vi "display language.vi"(6 "Language":T1, 8 "error in":errorcluster, 10 "Language data":T2=[{"Label.Text"="Quit", "Control Type"=0, "Numeric"=0.0, "Array"=[], "status"=FALSE, "Str Array"=[], "String"="", "unit"=""}, {"Label.Text"="Tab Control", "Control Type"=0, "Numeric"=0.0, "Array"=[], "status"=FALSE, "Str Array"=[], "String"="", "unit"=""}, {"Label.Text"="Help Button", "Control Type"=0, "Numeric"=0.0, "Array"=[], "status"=FALSE, "Str Array"=[], "String"="", "unit"=""}, {"Label.Text"="Logon", "Control Type"=0, "Numeric"=0.0, "Array"=[], "status"=FALSE, "Str Array"=[], "String"="", "unit"=""}, {"Label.Text"="Project List", "Control Type"=0, "Numeric"=0.0, "Array"=[], "status"=FALSE, "Str Array"=[], "String"="", "unit"=""}, {"Label.Text"="Project commands", "Control Type"=0, "Numeric"=0.0, "Array"=[], "status"=FALSE, "Str Array"=[], "String"="", "unit"=""}, {"Label.Text"="Log off", "Control Type"=0, "Numeric"=0.0, "Array"=[], "status"=FALSE, "Str Array"=[], "String"="", "unit"=""}, {"Label.Text"="Design Plant", "Control Type"=0, "Numeric"=0.0, "Array"=[], "status"=FALSE, "Str Array"=[], "String"="", "unit"=""}, {"Label.Text"="Project Info label", "Control Type"=0, "Numeric"=0.0, "Array"=[], "status"=FALSE, "Str Array"=[], "String"="", "unit"=""}, {"Label.Text"="Design Inputs Label", "Control Type"=0, "Numeric"=0.0, "Array"=[], "status"=FALSE, "Str Array"=[], "String"="", "unit"=""}, {"Label.Text"="MSG Design sent precity", "Control Type"=0, "Numeric"=0.0, "Array"=[], "status"=FALSE, "Str Array"=[], "String"="", "unit"=""}, {"Label.Text"="MSG Design sent postcity", "Control Type"=0, "Numeric"=0.0, "Array"=[], "status"=FALSE, "Str Array"=[], "String"="", "unit"=""}, {"Label.Text"="MSG Server unavailable", "Control Type"=0, "Numeric"=0.0, "Array"=[], "status"=FALSE, "Str Array"=[], "String"="", "unit"=""}, {"Label.Text"="Quit now", "Control Type"=0, "Numeric"=0.0, "Array"=[], "status"=FALSE, "Str Array"=[], "String"="", "unit"=""}, {"Label.Text"="Project Info", "Control Type"=0, "Numeric"=0.0, "Array"=[], "status"=FALSE, "Str Array"=[], "String"="", "unit"=""}, {"Label.Text"="Project Name", "Control Type"=0, "Numeric"=0.0, "Array"=[], "status"=FALSE, "Str Array"=[], "String"="", "unit"=""}, {"Label.Text"="City", "Control Type"=0, "Numeric"=0.0, "Array"=[], "status"=FALSE, "Str Array"=[], "String"="", "unit"=""}, {"Label.Text"="State", "Control Type"=0, "Numeric"=0.0, "Array"=[], "status"=FALSE, "Str Array"=[], "String"="", "unit"=""}, {"Label.Text"="Country", "Control Type"=0, "Numeric"=0.0, "Array"=[], "status"=FALSE, "Str Array"=[], "String"="", "unit"=""}, {"Label.Text"="Notes", "Control Type"=0, "Numeric"=0.0, "Array"=[], "status"=FALSE, "Str Array"=[], "String"="", "unit"=""}, {"Label.Text"="User Information", "Control Type"=0, "Numeric"=0.0, "Array"=[], "status"=FALSE, "Str Array"=[], "String"="", "unit"=""}, {"Label.Text"="First Name", "Control Type"=0, "Numeric"=0.0, "Array"=[], "status"=FALSE, "Str Array"=[], "String"="", "unit"=""}, {"Label.Text"="Last Name", "Control Type"=0, "Numeric"=0.0, "Array"=[], "status"=FALSE, "Str Array"=[], "String"="", "unit"=""}, {"Label.Text"="Email Address", "Control Type"=0, "Numeric"=0.0, "Array"=[], "status"=FALSE, "Str Array"=[], "String"="", "unit"=""}, {"Label.Text"="Organization", "Control Type"=0, "Numeric"=0.0, "Array"=[], "status"=FALSE, "Str Array"=[], "String"="", "unit"=""}, {"Label.Text"="Language", "Control Type"=0, "Numeric"=0.0, "Array"=[], "status"=FALSE, "Str Array"=[], "String"="", "unit"=""}, {"Label.Text"="AutoCAD File Type", "Control Type"=0, "Numeric"=0.0, "Array"=[], "status"=FALSE, "Str Array"=[], "String"="", "unit"=""}, {"Label.Text"="Project date", "Control Type"=0, "Numeric"=0.0, "Array"=[], "status"=FALSE, "Str Array"=[], "String"="", "unit"=""}, {"Label.Text"="Design Inputs", "Control Type"=0, "Numeric"=0.0, "Array"=[], "status"=FALSE, "Str Array"=[], "String"="", "unit"=""}, {"Label.Text"="Q.Plant", "Control Type"=0, "Numeric"=0.0, "Array"=[], "status"=FALSE, "Str Array"=[], "String"="", "unit"=""}, {"Label.Text"="C.CoagDoseMax", "Control Type"=0, "Numeric"=0.0, "Array"=[], "status"=FALSE, "Str Array"=[], "String"="", "unit"=""}, {"Label.Text"="C.CoagStock", "Control Type"=0, "Numeric"=0.0, "Array"=[], "status"=FALSE, "Str Array"=[], "String"="", "unit"=""}, {"Label.Text"="Ti.CoagStock", "Control Type"=0, "Numeric"=0.0, "Array"=[], "status"=FALSE, "Str Array"=[], "String"="", "unit"=""}, {"Label.Text"="EN.DrillSeries", "Control Type"=0, "Numeric"=0.0, "Array"=[], "status"=FALSE, "Str Array"=[], "String"="", "unit"=""}, {"Label.Text"="EN.TubeSeries", "Control Type"=0, "Numeric"=0.0, "Array"=[], "status"=FALSE, "Str Array"=[], "String"="", "unit"=""}, {"Label.Text"="EN.PipeSeries", "Control Type"=0, "Numeric"=0.0, "Array"=[], "status"=FALSE, "Str Array"=[], "String"="", "unit"=""}, {"Label.Text"="N.SedTanks", "Control Type"=0, "Numeric"=0.0, "Array"=[], "status"=FALSE, "Str Array"=[], "String"="", "unit"=""}, {"Label.Text"="N.SedBaysEst", "Control Type"=0, "Numeric"=0.0, "Array"=[], "status"=FALSE, "Str Array"=[], "String"="", "unit"=""}, {"Label.Text"="W.SedPlate", "Control Type"=0, "Numeric"=0.0, "Array"=[], "status"=FALSE, "Str Array"=[], "String"="", "unit"=""}, {"Label.Text"="L.SedPlateSheet", "Control Type"=0, "Numeric"=0.0, "Array"=[], "status"=FALSE, "Str Array"=[], "String"="", "unit"=""}, {"Label.Text"="T.SedPlate", "Control Type"=0, "Numeric"=0.0, "Array"=[], "status"=FALSE, "Str Array"=[], "String"="", "unit"=""}, {"Label.Text"="T.PlantWall", "Control Type"=0, "Numeric"=0.0, "Array"=[], "status"=FALSE, "Str Array"=[], "String"="", "unit"=""}, {"Label.Text"="H.FlocOption", "Control Type"=0, "Numeric"=0.0, "Array"=[], "status"=FALSE, "Str Array"=[], "String"="", "unit"=""}, {"Label.Text"="T.FlocBaffleRigidH", "Control Type"=0, "Numeric"=0.0, "Array"=[], "status"=FALSE, "Str Array"=[], "String"="", "unit"=""}, {"Label.Text"="T.ConcreteMin", "Control Type"=0, "Numeric"=0.0, "Array"=[], "status"=FALSE, "Str Array"=[], "String"="", "unit"=""}, {"Label.Text"="T.SedWeir", "Control Type"=0, "Numeric"=0.0, "Array"=[], "status"=FALSE, "Str Array"=[], "String"="", "unit"=""}, {"Label.Text"="T.FlocBaffleRigidV", "Control Type"=0, "Numeric"=0.0, "Array"=[], "status"=FALSE, "Str Array"=[], "String"="", "unit"=""}, {"Label.Text"="error out", "Control Type"=0, "Numeric"=0.0, "Array"=[], "status"=FALSE, "Str Array"=[], "String"="", "unit"=""}, {"Label.Text"="status", "Control Type"=0, "Numeric"=0.0, "Array"=[], "status"=FALSE, "Str Array"=[], "String"="", "unit"=""}, {"Label.Text"="code", "Control Type"=0, "Numeric"=0.0, "Array"=[], "status"=FALSE, "Str Array"=[], "String"="", "unit"=""}, {"Label.Text"="source", "Control Type"=0, "Numeric"=0.0, "Array"=[], "status"=FALSE, "Str Array"=[], "String"="", "unit"=""}, {"Label.Text"="File List", "Control Type"=0, "Numeric"=0.0, "Array"=[], "status"=FALSE, "Str Array"=[], "String"="", "unit"=""}, {"Label.Text"="Translate", "Control Type"=0, "Numeric"=0.0, "Array"=[], "status"=FALSE, "Str Array"=[], "String"="", "unit"=""}, {"Label.Text"="CheckOut ADT", "Control Type"=0, "Numeric"=0.0, "Array"=[], "status"=FALSE, "Str Array"=[], "String"="", "unit"=""}, {"Label.Text"="ADT version", "Control Type"=0, "Numeric"=0.0, "Array"=[], "status"=FALSE, "Str Array"=[], "String"="", "unit"=""}, {"Label.Text"="Choose Server", "Control Type"=0, "Numeric"=0.0, "Array"=[], "status"=FALSE, "Str Array"=[], "String"="", "unit"=""}, {"Label.Text"="design server", "Control Type"=0, "Numeric"=0.0, "Array"=[], "status"=FALSE, "Str Array"=[], "String"="", "unit"=""}, {"Label.Text"="Restart ADT", "Control Type"=0, "Numeric"=0.0, "Array"=[], "status"=FALSE, "Str Array"=[], "String"="", "unit"=""}, {"Label.Text"="Create New Project", "Control Type"=0, "Numeric"=0.0, "Array"=[], "status"=FALSE, "Str Array"=[], "String"="", "unit"=""}, {"Label.Text"="Edit Project", "Control Type"=0, "Numeric"=0.0, "Array"=[], "status"=FALSE, "Str Array"=[], "String"="", "unit"=""}, {"Label.Text"="Delete Project", "Control Type"=0, "Numeric"=0.0, "Array"=[], "status"=FALSE, "Str Array"=[], "String"="", "unit"=""}, {"Label.Text"="Valid User Options", "Control Type"=0, "Numeric"=0.0, "Array"=[], "status"=FALSE, "Str Array"=[], "String"="", "unit"=""}, {"Label.Text"="Okay Button", "Control Type"=0, "Numeric"=0.0, "Array"=[], "status"=FALSE, "Str Array"=[], "String"="", "unit"=""}, {"Label.Text"="logon status", "Control Type"=0, "Numeric"=0.0, "Array"=[], "status"=FALSE, "Str Array"=[], "String"="", "unit"=""}, {"Label.Text"="valid user", "Control Type"=0, "Numeric"=0.0, "Array"=[], "status"=FALSE, "Str Array"=[], "String"="", "unit"=""}, {"Label.Text"="User Information out", "Control Type"=0, "Numeric"=0.0, "Array"=[], "status"=FALSE, "Str Array"=[], "String"="", "unit"=""}, {"Label.Text"="Cancel Button", "Control Type"=0, "Numeric"=0.0, "Array"=[], "status"=FALSE, "Str Array"=[], "String"="", "unit"=""}, {"Label.Text"="User Index out", "Control Type"=0, "Numeric"=0.0, "Array"=[], "status"=FALSE, "Str Array"=[], "String"="", "unit"=""}, {"Label.Text"="User Index in", "Control Type"=0, "Numeric"=0.0, "Array"=[], "status"=FALSE, "Str Array"=[], "String"="", "unit"=""}, {"Label.Text"="New Account", "Control Type"=0, "Numeric"=0.0, "Array"=[], "status"=FALSE, "Str Array"=[], "String"="", "unit"=""}, {"Label.Text"="Update User Info", "Control Type"=0, "Numeric"=0.0, "Array"=[], "status"=FALSE, "Str Array"=[], "String"="", "unit"=""}, {"Label.Text"="Language Data", "Control Type"=0, "Numeric"=0.0, "Array"=[], "status"=FALSE, "Str Array"=[], "String"="", "unit"=""}, {"Label.Text"="OK Button", "Control Type"=0, "Numeric"=0.0, "Array"=[], "status"=FALSE, "Str Array"=[], "String"="", "unit"=""}, {"Label.Text"="Language Data out", "Control Type"=0, "Numeric"=0.0, "Array"=[], "status"=FALSE, "Str Array"=[], "String"="", "unit"=""}, {"Label.Text"="updated", "Control Type"=0, "Numeric"=0.0, "Array"=[], "status"=FALSE, "Str Array"=[], "String"="", "unit"=""}, {"Label.Text"="Table Control", "Control Type"=0, "Numeric"=0.0, "Array"=[], "status"=FALSE, "Str Array"=[], "String"="", "unit"=""}, {"Label.Text"="Load from VNG", "Control Type"=0, "Numeric"=0.0, "Array"=[], "status"=FALSE, "Str Array"=[], "String"="", "unit"=""}, {"Label.Text"="Design Inputs out", "Control Type"=0, "Numeric"=0.0, "Array"=[], "status"=FALSE, "Str Array"=[], "String"="", "unit"=""}, {"Label.Text"="Project Info out", "Control Type"=0, "Numeric"=0.0, "Array"=[], "status"=FALSE, "Str Array"=[], "String"="", "unit"=""}, {"Label.Text"="canceled", "Control Type"=0, "Numeric"=0.0, "Array"=[], "status"=FALSE, "Str Array"=[], "String"="", "unit"=""}, {"Label.Text"="Reset to Default", "Control Type"=0, "Numeric"=0.0, "Array"=[], "status"=FALSE, "Str Array"=[], "String"="", "unit"=""}, {"Label.Text"="Basic Inputs", "Control Type"=0, "Numeric"=0.0, "Array"=[], "status"=FALSE, "Str Array"=[], "String"="", "unit"=""}, {"Label.Text"="Floc tank depth controls", "Control Type"=0, "Numeric"=0.0, "Array"=[], "status"=FALSE, "Str Array"=[], "String"="", "unit"=""}, {"Label.Text"="HW.FlocEnd", "Control Type"=0, "Numeric"=0.0, "Array"=[], "status"=FALSE, "Str Array"=[], "String"="", "unit"=""}, {"Label.Text"="HW.FlocEndDepth", "Control Type"=0, "Numeric"=0.0, "Array"=[], "status"=FALSE, "Str Array"=[], "String"="", "unit"=""}, {"Label.Text"="Language data", "Control Type"=0, "Numeric"=0.0, "Array"=[], "status"=FALSE, "Str Array"=[], "String"="", "unit"=""}, {"Label.Text"="error in", "Control Type"=0, "Numeric"=0.0, "Array"=[], "status"=FALSE, "Str Array"=[], "String"="", "unit"=""}, {"Label.Text"="VI controls", "Control Type"=0, "Numeric"=0.0, "Array"=[], "status"=FALSE, "Str Array"=[], "String"="", "unit"=""}, {"Label.Text"="Progress bar", "Control Type"=0, "Numeric"=0.0, "Array"=[], "status"=FALSE, "Str Array"=[], "String"="", "unit"=""}], 11 "VI controls":refnum<vi>[](array[refnum])) -> (0 "error out":errorcluster)   [LabVIEW 2015, in "AguaClara Library.lvlib"]
uses:
  AguaClara Library.lvlib
  Language.ctl
  Variable cluster.ctl
panel:
  out "Control labels":string[](array[string])
  out "Progress bar":dbl(slide) caption="Traduciendo" max=314.0 scale=0.0..1.0
  in  "Cancel Button":bool caption="Cancelar"
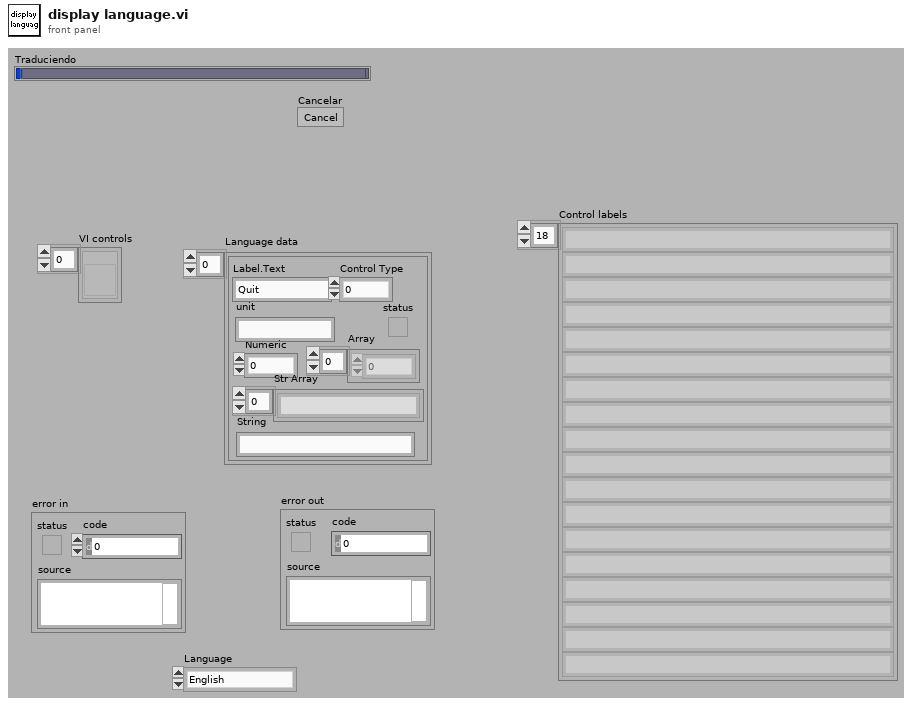
[diagram p1: front panel]
types:
  T1 = typedef "AguaClara Library.lvlib/Language.ctl" = enum16{"English", "Español", "French"}
  T2 = typedef "Variable cluster.ctl" = cluster{"Label.Text":string, "Control Type":u32, "Numeric":dbl, "Array":dbl[], "status":bool, "Str Array":string[], "String":string, "unit":string}[]
  T3 = cluster{"Label.Text":string, "Control Type":u32, "Numeric":dbl, "Array":dbl[], "status":bool, "Str Array":string[], "String":string, "unit":string}
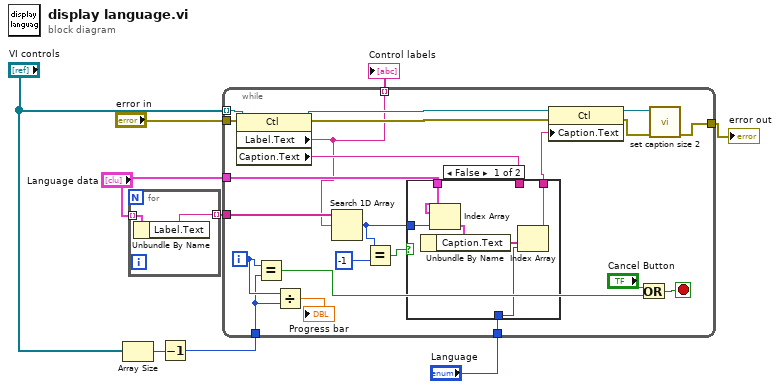
[diagram p0: block diagram]
diagram:
  n1 = Array Size(array="VI controls") -> (size(s)=w3:i32)
  n2 = for {
    tunnel: "Language data" -> [w11] mode=indexing
    tunnel: [w10] -> w5 mode=indexing
    n3 = Unbundle By Name(w11) -> ("Label.Text"=w10:string)
  }
  n4 = Decrement(x=w3) -> (x-1=w2:i32)
  n5 = while {
    tunnel: "VI controls" -> [w33] mode=indexing
    tunnel: "error in" -> [w32]
    tunnel: w5 -> [w30]
    tunnel: "Language data" -> [w29]
    tunnel: [w19] -> w6
    tunnel: "Language" -> [w28]
    tunnel: w2 -> [w17]
    tunnel: [w12] -> w1 mode=indexing
    i -> [w18]
    stop <- w13 stop-if-true
    n6 = property class="Ctl"(reference=w33, error in=w32) -> (reference out=w31:refnum<vi>, error out=w24:errorcluster, "Label.Text"=w12:string, "Caption.Text"=w23:string)
    n7 = Equal?(x=w18, y=w17) -> (x = y?=w14:bool)
    n8 = Divide(x=w18, y=w17) -> (x/y=→"Progress bar":dbl)
    n9 = Search 1D Array(1D array=w30, element=w12) -> (index of element=w27:i32)  [unwired: 1 in]
    n10 = Equal?(x=w27, y=-1) -> (x = y?=w25:bool)
    n11 = case shown="False" w25 {
      tunnel: w27 -> [w39 _]
      tunnel: w29 -> [w35 _]
      tunnel: [w37 w40] -> w22
      tunnel: w28 -> [w36 _]
      tunnel: w23 -> [_ w40]
      frame False {
        n12 = Index Array(array=w35, index=w39) -> (element=w34:T3)
        n13 = Unbundle By Name(w34) -> ("Caption.Text"=w38:string[])
        n14 = Index Array(array=w38, index=w36) -> (element=w37:string)
      }
      frame True {
      }
    }
    n15 = property class="Ctl"(reference=w31, error in=w24, "Caption.Text"=w22) -> (reference out=w21:refnum<vi>, error out=w20:errorcluster)
    n16 = Or(x="Cancel Button", y=w14) -> (x .or. y?=w13:bool)
    n17 = call "set caption size 2.vi"("error in (no error)"=w20, "Ctl Refnum in"=w21) -> ("error out"=w19:errorcluster)  [unwired: 8 in, 1 out]
  }
  "error out" <- w6
  "Control labels" <- w1
